vi "test realtime main (no data).vi"() -> ()   [LabVIEW 2012]
panel:
  in  "Display Trace Offset":dbl
  in  "output cluster":T1
  out "Z2":dbl[][](graph)
  out "Y2":dbl[][](graph)
  out "X2":dbl[][](graph)
  out "Z1":dbl[][](graph)
  out "Y1":dbl[][](graph)
  out "X1":dbl[][](graph)
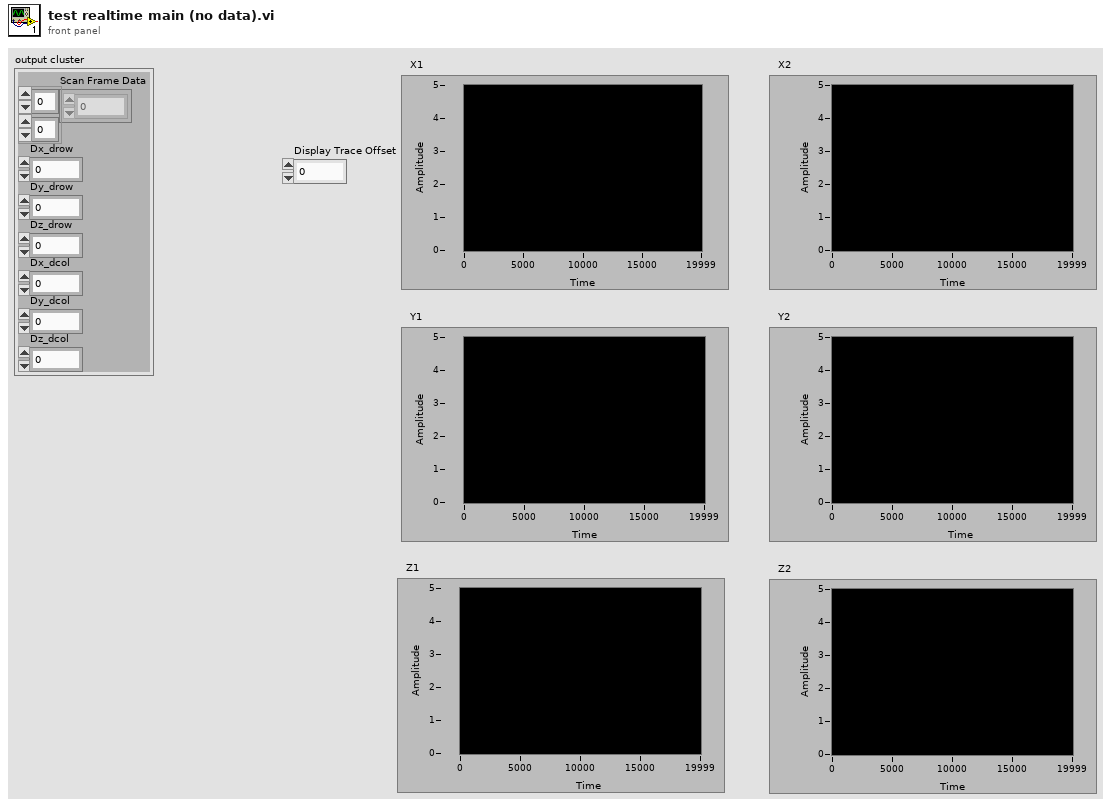
[diagram p1: front panel]
types:
  T1 = cluster{"Scan Frame Data":dbl[][], "Dx_drow":dbl, "Dy_drow":dbl, "Dz_drow":dbl, "Dx_dcol":dbl, "Dy_dcol":dbl, "Dz_dcol":dbl}
  T2 = cluster{"PMTChans":i32, "NumScanPlanes":i32, "ScanRows":i32, "ScanCols":i32, "NumSamples":i32}
  T3 = cluster{"Scan Frame Data":dbl[][], "Dx_drow":dbl, "Dy_drow":dbl, "Dz_drow":dbl, "Dx_dcol":dbl, "Dy_dcol":dbl, "Dz_dcol":dbl}[]
  T4 = cluster{"Scan Frame Data":dbl[][], dbl, dbl, dbl, dbl, dbl, dbl}
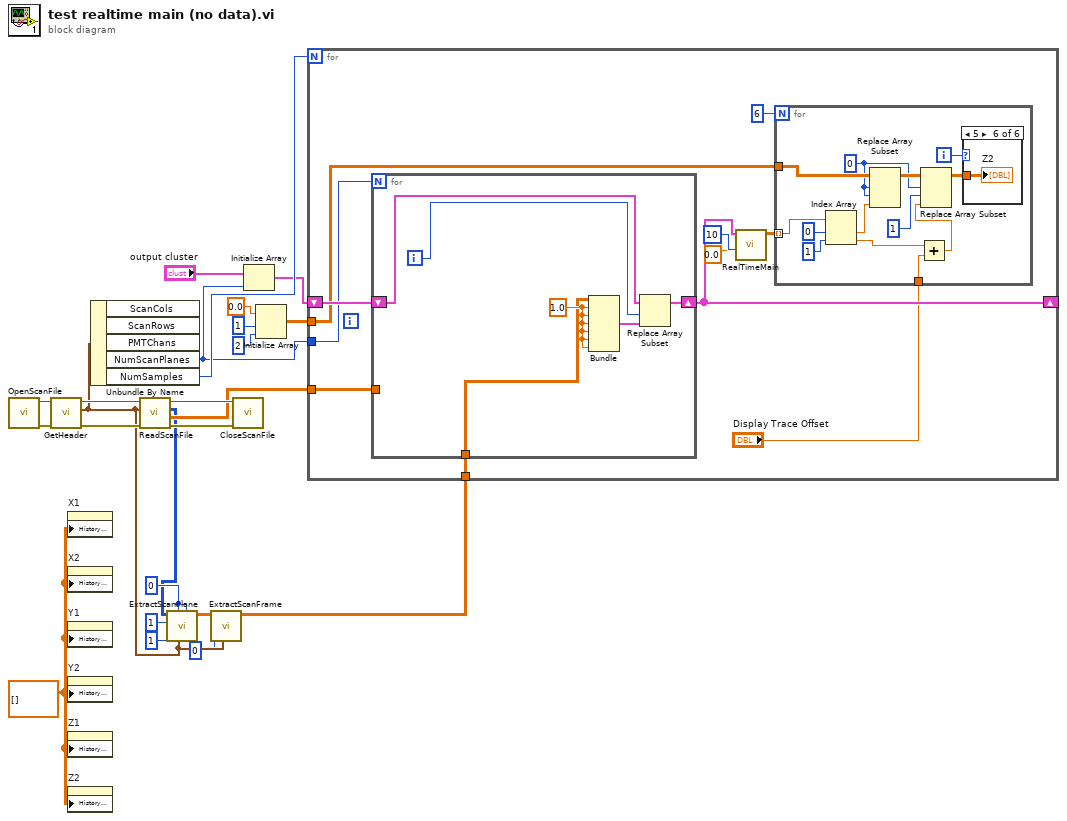
[diagram p0: block diagram]
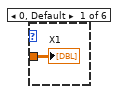
[diagram p2: hidden frame]
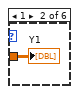
[diagram p3: hidden frame]
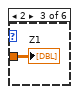
[diagram p4: hidden frame]
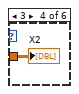
[diagram p5: hidden frame]
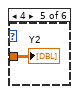
[diagram p6: hidden frame]
diagram:
  w8 = 0 ("Start Frame")
  w9 = dbl[][] [] ("History Data")
  n1 = call "OpenScanFile.vi"() -> ("error out"=w23:errorcluster, "refnum out"=w24:refnum<file>)  [unwired: 10 in]
  n2 = call "GetHeader.vi"("error in"=w23, "refnum in"=w24) -> ("error out"=w19:errorcluster, "Header"=w4:T2, "refnum out"=w22:refnum<file>)  [unwired: 6 in]
  n3 = property on="X1" class="WFChart (strict)"("History Data"=w9) -> ()  [unwired: 2 in, 2 out]
  n4 = property on="X2" class="WFChart (strict)"("History Data"=w9) -> ()  [unwired: 2 in, 2 out]
  n5 = property on="Y1" class="WFChart (strict)"("History Data"=w9) -> ()  [unwired: 2 in, 2 out]
  n6 = property on="Y2" class="WFChart (strict)"("History Data"=w9) -> ()  [unwired: 2 in, 2 out]
  n7 = property on="Z1" class="WFChart (strict)"("History Data"=w9) -> ()  [unwired: 2 in, 2 out]
  n8 = property on="Z2" class="WFChart (strict)"("History Data"=w9) -> ()  [unwired: 2 in, 2 out]
  n9 = Unbundle By Name(w4) -> ("NumScanPlanes"=w15:i32, "NumSamples"=w17:i32)  [unwired: 3 out]
  n10 = call "ReadScanFile.vi"("error in"=w19, "Header"=w4, "refnum in"=w22) -> ("error out"=w20:errorcluster, "Coordinate Data"=w18:dbl[][][][], "Scan Data"=w7:i32[][][][], "refnum out"=w21:refnum<file>)  [unwired: 5 in]
  n11 = call "ExtractScanPlane.vi"("End Frame"=w8, "Header"=w4, "Start Frame"=w8, "Scan Plane"=1, "PMT Channel"=1, "All Scan Data"=w7) -> ("Scan Plane Data"=w3:dbl[][][])  [unwired: 5 in]
  n12 = call "ExtractScanFrame.vi"("Header"=w4, "Scan Frame"=0, "Scan Plane Data"=w3) -> ("Scan Frame Data"=w1:dbl[][])  [unwired: 8 in]
  n13 = call "CloseScanFile.vi"("error in"=w20, "refnum"=w21) -> ()  [unwired: 9 in, 1 out]
  n14 = Initialize Array("output cluster", w15) -> (w14:T3)
  n15 = Initialize Array(0.0 ("element"), 1 ("dimension size"), 2 ("dimension size")) -> (w10:dbl[][])
  n16 = for {
    N: w17 -> [_]
    tunnel: w18 -> [w35]
    tunnel: w15 -> [w33]
    shift-right: [w30] -> _
    shift-left: w14 -> [w34]
    tunnel: w10 -> [w31]
    tunnel: w1 -> [w26]
    n17 = for {
      N: w33 -> [_]
      tunnel: w35 -> [_]
      shift-right: [w57] -> w30
      shift-left: w34 -> [w60]
      tunnel: w26 -> [w55]
      i -> [w58]
      w56 = 1.0
      n18 = Bundle("Scan Frame Data"=w55, w56, w56, w56, w56, w56, w56) -> (w59:T4)  [unwired: 1 in]
      n19 = Replace Array Subset(array=w60, new element=w59, index=w58) -> (w57:T3)
    }
    n20 = call "RealTimeMain.vi"(8:0.0 ("Threshold (microns)"), "For Reference (frames)"=10, "Motion Data"=w30) -> ("Array"=w27:dbl[][])  [unwired: 8 in]
    n21 = for {
      N: 6 -> [_]
      tunnel: w31 -> [w45]
      tunnel: w27 -> [w40] mode=indexing
      tunnel: "Display Trace Offset" -> [w36]
      i -> [w48]
      w42 = 0 ("index")
      n22 = Index Array(array=w40, index #1=0 ("index"), index #2=1 ("index")) -> (element #1=w44:dbl, element #2=w37:dbl)
      n23 = Replace Array Subset(array=w45, new element=w44, index (row)=w42, index (col)=w42) -> (w43:dbl[][])
      n24 = Add(x=w37, y=w36) -> (x+y=w38:dbl)
      n25 = Replace Array Subset(array=w43, new element=w38, index (row)=w42, index (col)=1 ("disabled index (col)")) -> (w41:dbl[][])
      n26 = case shown="5" w48 {
        tunnel: w41 -> [w49 w50 w51 w52 w53 w54]
        frame 0, Default {
          "X1" <- w49
        }
        frame 1 {
          "Y1" <- w50
        }
        frame 2 {
          "Z1" <- w51
        }
        frame 3 {
          "X2" <- w52
        }
        frame 4 {
          "Y2" <- w53
        }
        frame 5 {
          "Z2" <- w54
        }
      }
    }
  }
